vi "Test lib template open.vi"() -> ()   [LabVIEW 2016]
panel:
  out "error out":errorcluster
  in  "error in (no error)":errorcluster
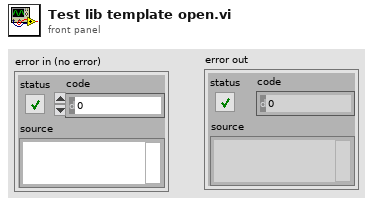
[diagram p1: front panel]
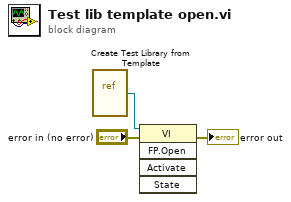
[diagram p0: block diagram]
diagram:
  n1 = vi-ref "Create Test Library from Template.vi"() -> (w3:refnum<vi>)
  n2 = invoke class="VI" method="FP.Open"(reference=w3, error in="error in (no error)") -> (error out=→"error out":errorcluster)  [unwired: 3 in, 4 out]
